vi "Revert Running Test Colors.vi"(8 "Error In":errorcluster, 10 "TopLevel in":T1, 11 "QSM In":string[](array[string])) -> (0 "Error Out":errorcluster, 2 "TopLevel out":T1, 3 "QSM out":string[](array[string]))   [LabVIEW 2011]
uses:
  Controls/Top Level Control.ctl
  <vilib>/NI/AMC/Message Queue.ctl
  <vilib>/NI/AMC/Message.ctl
  <vilib>/NI/Tools/Keyed Array/KeyedArray.ctl
  Controls/ListBox Test Record.ctl
  Controls/DVR of CSV Tests Data.ctl
  Controls/CSVs Tests Data.ctl
  Controls/Test Column Data.ctl
  Controls/Options DVR.ctl
  Controls/Options.ctl
  <vilib>/NI/Tools/Keyed Array/Tools_KeyedArray.lvlib
  <vilib>/NI/AMC/AMC.lvlib
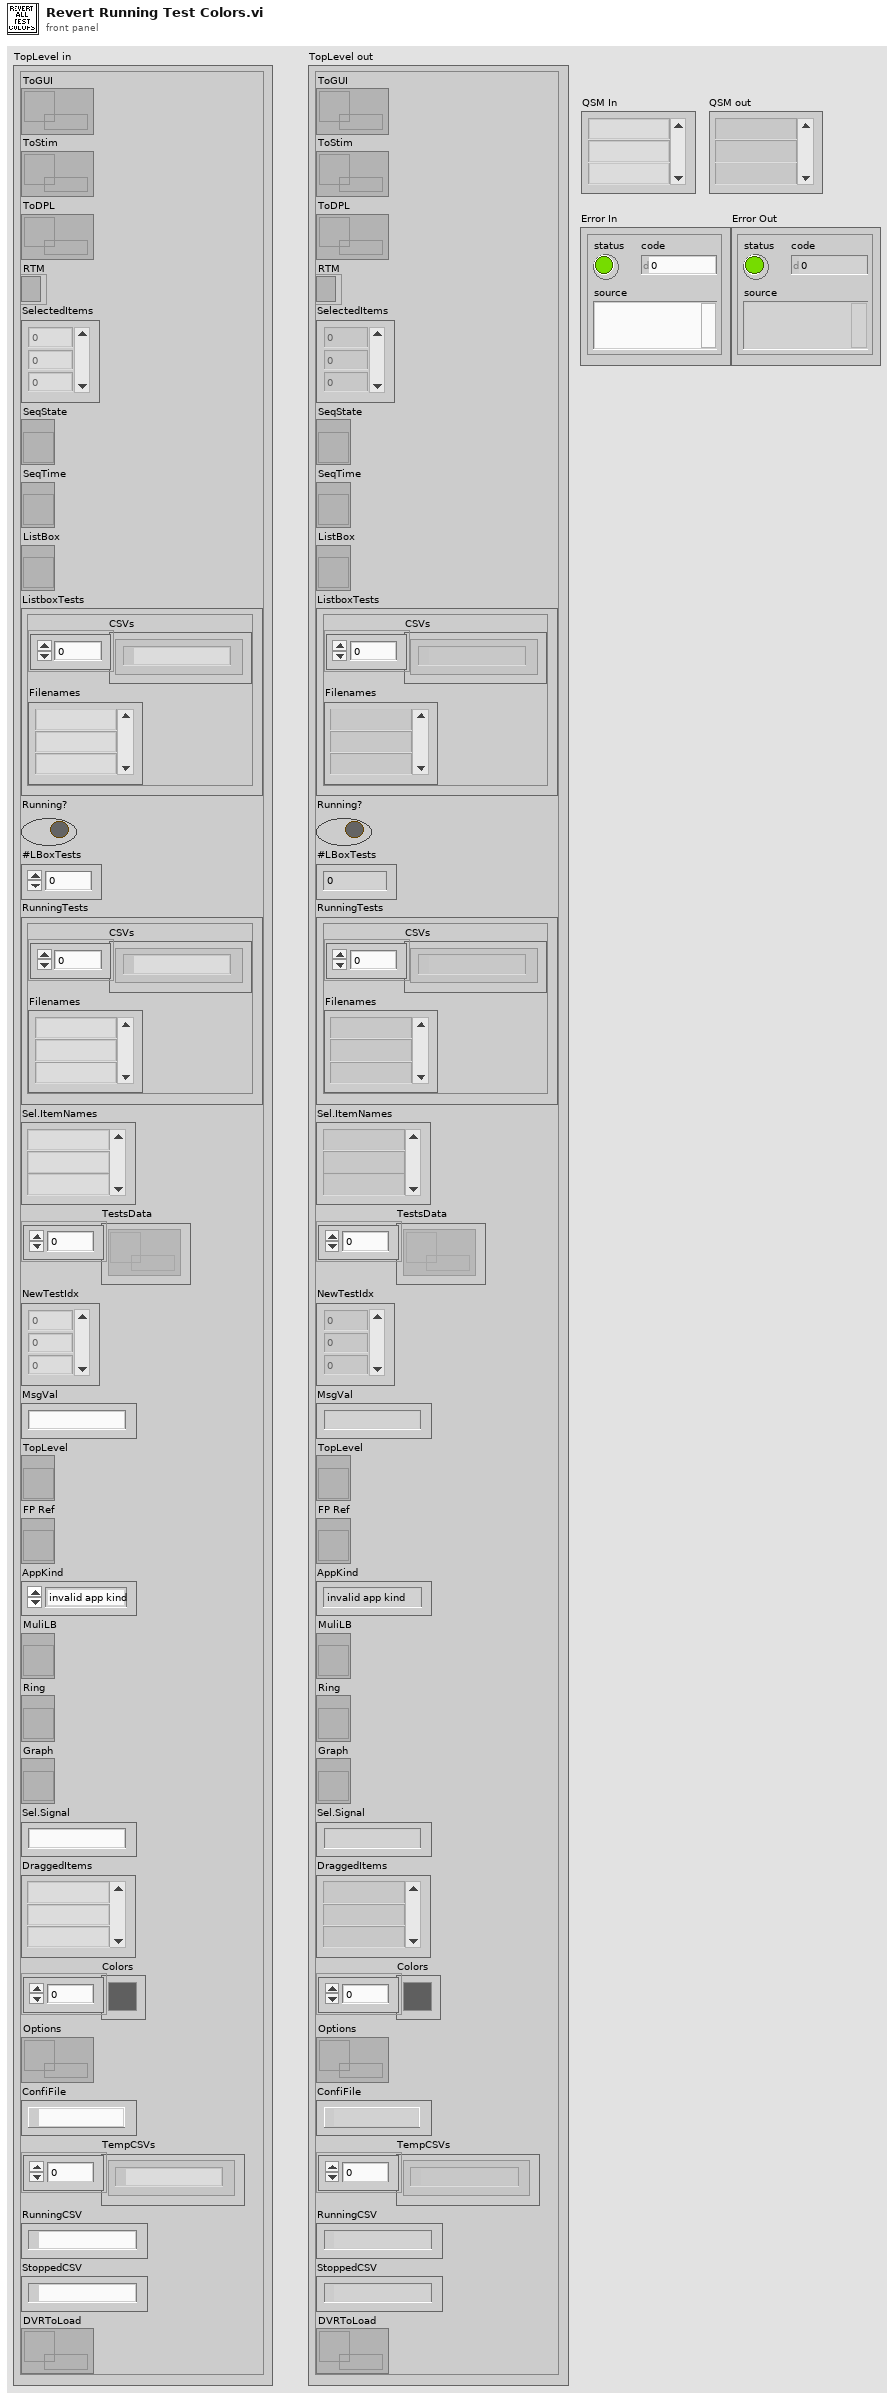
[diagram p1: front panel]
types:
  T1 = typedef "Top Level Control.ctl" = cluster{"ToGUI":T2, "ToStim":T2, "ToDPL":T2, "RTM":refnum<k9>, "SelectedItems":i32[], "SeqState":refnum<vi>, "SeqTime":refnum<vi>, "ListBox":refnum<vi>, "ListboxTests":T3, "Running?":bool, "#LBoxTests":i32, "RunningTests":T3, "Sel.ItemNames":string[], "TestsData":T4[], "NewTestIdx":i32[], "MsgVal":string, "TopLevel":refnum<vi>, "FP Ref":refnum<vi>, "AppKind":enum32{"invalid app kind", "Development System", "Run Time System", "Student Edition", "Embedded LabVIEW", "Evaluation", "Custom"}, "MuliLB":refnum<vi>, "Ring":refnum<vi>, "Graph":refnum<vi>, "Sel.Signal":string, "DraggedItems":string[], "Colors":u32[], "Options":T5, "ConfiFile":path, "TempCSVs":path[], "RunningCSV":path, "StoppedCSV":path, "DVRToLoad":T4}
  T2 = typedef "AMC.lvlib/Message Queue.ctl" = refnum<queue>
  T3 = typedef "ListBox Test Record.ctl" = cluster{"CSVs":path[], "Filenames":string[]}
  T4 = typedef "DVR of CSV Tests Data.ctl" = refnum<data-value>
  T5 = typedef "Options DVR.ctl" = refnum<data-value>
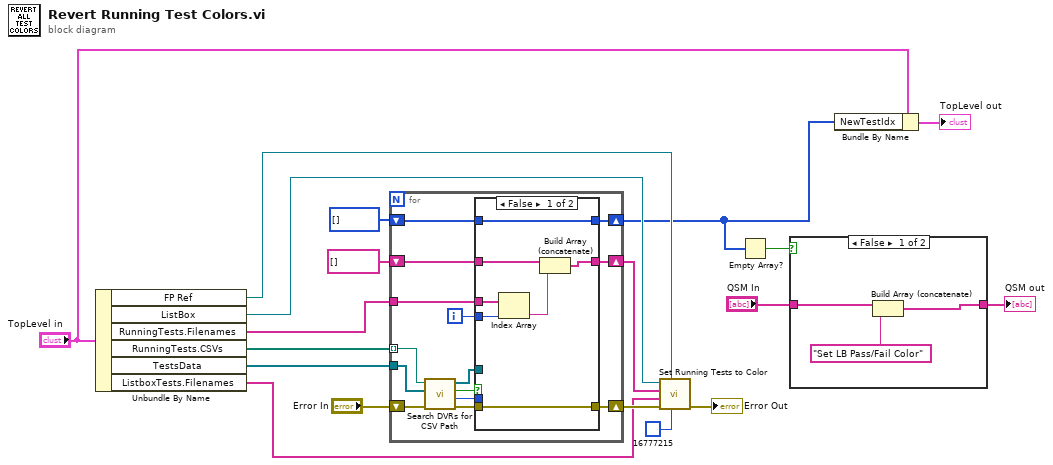
[diagram p0: block diagram]
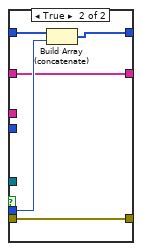
[diagram p3: hidden frame]
diagram:
  n1 = Unbundle By Name("TopLevel in") -> ("FP Ref"=w10:refnum<vi>, "ListBox"=w9:refnum<vi>, "RunningTests.Filenames"=w14:string[], "RunningTests.CSVs"=w19:path[], "TestsData"=w18:T4[], "ListboxTests.Filenames"=w12:string[])
  n2 = for {
    tunnel: w19 -> [w32] mode=indexing
    tunnel: w18 -> [w31]
    shift-right: [w24] -> w13
    shift-left: "Error In" -> [w33]
    shift-right: [w25] -> w4
    shift-left: i32[] [] -> [w26]
    shift-right: [w23] -> w11
    shift-left: string[] [] -> [w22]
    tunnel: w14 -> [w21]
    i -> [w20]
    n3 = call "Search DVRs for CSV Path.vi"("error in (no error)"=w33, "DVRs"=w31, "CsvPath"=w32) -> ("error out"=w29:errorcluster, "Idx"=w27:i32, "Found?"=w30:bool, "DVRs dup"=w28:T4[])  [unwired: 5 in]
    n4 = case shown="False" w30 {
      tunnel: w29 -> [w34 w42]
      tunnel: w28 -> [_ _]
      tunnel: w27 -> [_ w44]
      tunnel: w26 -> [w40 w45]
      tunnel: [w40 w43] -> w25
      tunnel: [w34 w42] -> w24
      tunnel: [w38 w41] -> w23
      tunnel: w22 -> [w39 w41]
      tunnel: w21 -> [w37 _]
      tunnel: w20 -> [w36 _]
      frame False {
        n5 = Index Array(array=w37, index=w36) -> (element=w35:string)
        n6 = Build Array (concatenate)(w39, w35) -> (w38:string[])
      }
      frame True {
        n7 = Build Array (concatenate)(w45, w44) -> (w43:i32[])
      }
    }
  }
  n8 = call "Set Running Tests to Color.vi"("Color"=u32 16777215, "FP Ref"=w10, "Error In"=w13, "Listbox Tests"=w12, "Running Tests"=w11, "Tests"=w9) -> ("Error Out"=→"Error Out":errorcluster)  [unwired: 5 in]
  n9 = Empty Array?(array=w4) -> (empty?=w3:bool)
  n10 = case shown="False" w3 {
    tunnel: [w47 w49] -> w1
    tunnel: "QSM In" -> [w48 w49]
    frame False {
      n11 = Build Array (concatenate)(w48, "Set LB Pass/Fail Color") -> (w47:string[])
    }
    frame True {
    }
  }
  "QSM out" <- w1
  n12 = Bundle By Name(cluster="TopLevel in", "NewTestIdx"=w4) -> (→"TopLevel out":T1)
